vi "Heartbeat.vi"(1 "Loop Iteration":i32) -> (0 "Running?":bool)   [LabVIEW 2010]
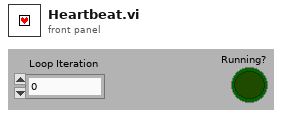
[diagram p1: front panel]
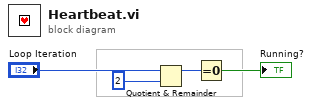
[diagram p0: block diagram]
diagram:
  n1 = Quotient & Remainder(x="Loop Iteration", y=2) -> (x-y*floor(x/y)=w3:i32)  [unwired: 1 out]
  n2 = Equal To 0?(x=w3) -> (x = 0?=→"Running?":bool)
